vi "Create Object (drawable with reference).vi"(8 "error in (no error)":errorcluster, 10 "Geometry or text":refnum<vi>, 11 "Name":string) -> (0 "error out":errorcluster, 2 "Drawable refnum":refnum<vi>, 3 "Scene:New Object":refnum<vi>)   [LabVIEW 2020, in "NI_3D Picture Control.lvlib"]
doc: "Creates a new 3D object to display in the 3D scene."
uses:
  <vilib>/picture/3D Picture Control/NI_3D Picture Control.lvlib
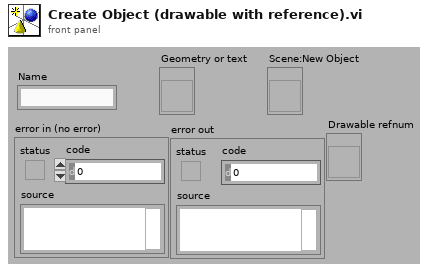
[diagram p1: front panel]
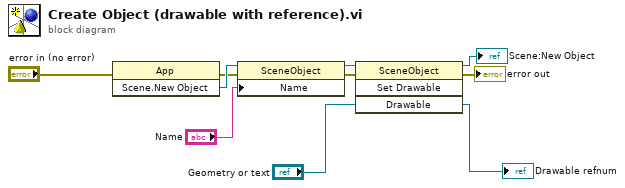
[diagram p0: block diagram]
diagram:
  n1 = invoke class="App" method="Scene.New Object"(error in="error in (no error)") -> (error out=w8:errorcluster, "Scene.New Object"=w9:refnum<vi>)  [unwired: 2 in, 1 out]
  n2 = property class="SceneObject"(reference=w9, error in=w8, "Name"="Name") -> (reference out=w6:refnum<vi>, error out=w5:errorcluster)
  n3 = invoke class="SceneObject" method="Set Drawable"(reference=w6, error in=w5, "Drawable"="Geometry or text") -> (reference out=→"Scene:New Object":refnum<vi>, error out=→"error out":errorcluster, "Drawable"=→"Drawable refnum":refnum<vi>)  [unwired: 1 in, 1 out]
